vi "Test - Refnum Subtype Enum.vi"() -> ()   [LabVIEW 2020]
uses:
  source/library/oglib_lvdata.lvlib
  source/library/Refnum Subtype Enum.ctl
panel:
  out "30 LabVIEW Class":T1 format="%.0x"
  out "31 Data Value Refnum":T1 format="%.0x"
  out "21 HPT Refnum: Shared Variable Refnum":T1 format="%.0x"
  out "34 TDMS Refnum":T1 format="%.0x"
  out "25 User Event Refnum":T1 format="%.0x"
  out "23 Event Registration Refnum":T1 format="%.0x"
  out "18 Queue Refnum":T1 format="%.0x"
  out "17 Notifier Refnum":T1 format="%.0x"
  out "21 HPT Refnum: DAQmx Global Channel":T1 format="%.0x"
  out "21 HPT Refnum: FieldPoint IO Point":T1 format="%.0x"
  out "14 VISA resource name":T1 format="%.0x"
  out "15 IVI Logical Name":T1 format="%.0x"
  out "21 HPT Refnum: Motion Resource":T1 format="%.0x"
  out "11 IMAQ Session":T1 format="%.0x"
  in  "Motion Resource":refnum<k21>
  in  "FieldPoint IO Point":refnum<k21>
  out "08 VI Server Refnum":T1 format="%.0x"
  out "19 IrDA Refnum":T1 format="%.0x"
  out "31 Bluetooth Refnum":T1 format="%.0x"
  out "24 .NET Refnum":T1 format="%.0x"
  out "27 Event Callback Refnum":T1 format="%.0x"
  out "07 Automation Refnum":T1 format="%.0x"
  out "16 UDP Refnum":T1 format="%.0x"
  out "05 TCP Refnum":T1 format="%.0x"
  out "13 Datasocket Refnum":T1 format="%.0x"
  out "09 Menu Refnum":T1 format="%.0x"
  out "04 Occurence Refnum":T1 format="%.0x"
  out "02 Datalog File Refnum":T1 format="%.0x"
  out "01 Byte Stream File Refnum":T1 format="%.0x"
  out "00 Generic":T1 format="%.0x"
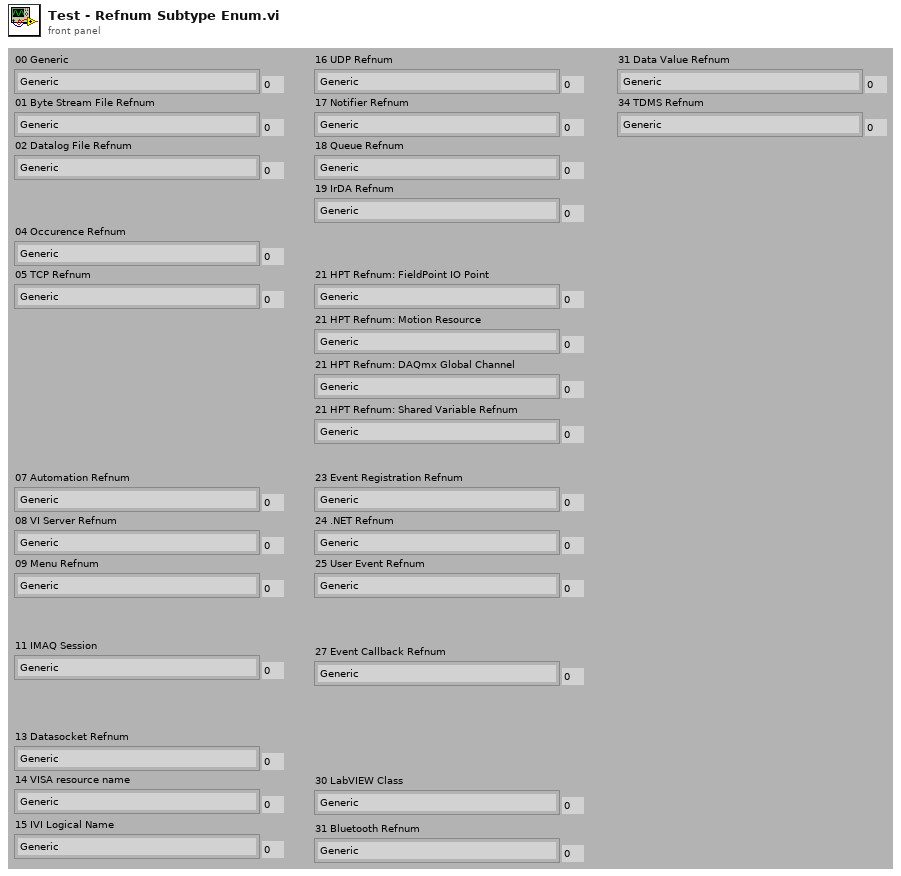
[diagram p1: front panel]
types:
  T1 = typedef "oglib_lvdata.lvlib/Refnum Subtype Enum.ctl" = enum8{"Generic", "Datalog File Refnum", "Byte Stream File Refnum", "Device Refnum", "Occurence Refnum", "TCP Connection Refnum", "VISA Refnum (Obsolete)", "Automation Renum", "VI Server Refnum", "Menu Refnum", "IVI Refnum (Obsolete)", "IMAQ Session", "0x0C", "Datasocket Refnum", "VISA Resource", "IVI Logical Name", "UDP Connection Refnum", "Notifier Refnum", "Queue Refnum", "IrDA Refnum", "Hardware Plugin Refnum", "Hardware Plugin Tag Refnum", "DAQmx Refnum", "Event Registration Refnum", ".NET Refnum", "User Event Refnum", "0x1A", "Event Callback", "0x1C", "0x1D", "LabVIEW Class Instance", "Bluetooth", "Data Value References", "RT FIFO", "TDM Streaming"}
  T2 = typedef "Refnum Subtype Enum.ctl" = enum8{"Generic", "Datalog File Refnum", "Byte Stream File Refnum", "Device Refnum", "Occurence Refnum", "TCP Connection Refnum", "VISA Refnum (Obsolete)", "Automation Renum", "VI Server Refnum", "Menu Refnum", "IVI Refnum (Obsolete)", "IMAQ Session", "0x0C", "Datasocket Refnum", "VISA Resource", "IVI Logical Name", "UDP Connection Refnum", "Notifier Refnum", "Queue Refnum", "IrDA Refnum", "Hardware Plugin Refnum", "Hardware Plugin Tag Refnum", "DAQmx Refnum", "Event Registration Refnum", ".NET Refnum", "User Event Refnum", "0x1A", "Event Callback", "0x1C", "0x1D", "LabVIEW Class Instance", "Bluetooth", "Data Value References", "RT FIFO", "TDM Streaming"}
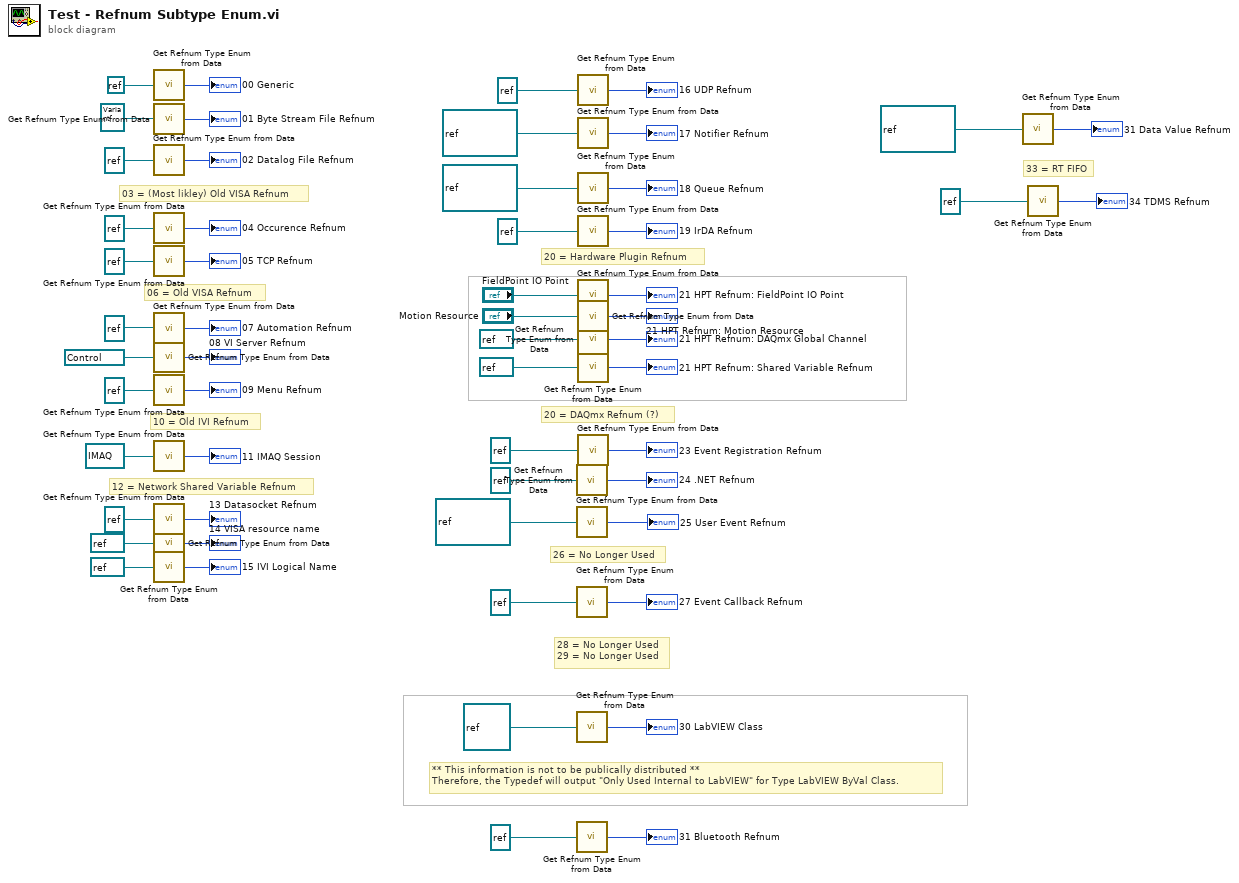
[diagram p0: block diagram]
diagram:
  # "20 = DAQmx Refnum (?)"
  # "20 = Hardware Plugin Refnum"
  # "28 = No Longer Used\n29 = No Longer Used"
  # "26 = No Longer Used"
  # "10 = Old IVI Refnum"
  # "06 = Old VISA Refnum"
  # "03 = (Most likley) Old VISA Refnum"
  # "12 = Network Shared Variable Refnum"
  # "33 = RT FIFO"
  # "** This information is not to be publically distributed **\nTherefore, the Typedef will output \"Only Used Internal to LabVIEW\" for Type LabVIEW ByVal Class."
  n1 = call "Get Refnum Type Enum from Data.vi"("Data"=refnum<k0> refnum) -> ("Refnum Subtype Enum"=→"00 Generic":T2)  [unwired: 4 in]
  n2 = call "Get Refnum Type Enum from Data.vi"("Data"=refnum<k1> refnum ("refnum out")) -> ("Refnum Subtype Enum"=→"01 Byte Stream File Refnum":T2)  [unwired: 4 in]
  n3 = call "Get Refnum Type Enum from Data.vi"("Data"=refnum<file> refnum ("refnum")) -> ("Refnum Subtype Enum"=→"02 Datalog File Refnum":T2)  [unwired: 4 in]
  n4 = call "Get Refnum Type Enum from Data.vi"("Data"=refnum<k4> refnum ("occurrence")) -> ("Refnum Subtype Enum"=→"04 Occurence Refnum":T2)  [unwired: 4 in]
  n5 = call "Get Refnum Type Enum from Data.vi"("Data"=refnum<k5> refnum ("TCP Network Connection Refnum")) -> ("Refnum Subtype Enum"=→"05 TCP Refnum":T2)  [unwired: 4 in]
  n6 = call "Get Refnum Type Enum from Data.vi"("Data"=refnum<k7> refnum ("Automation Refnum")) -> ("Refnum Subtype Enum"=→"07 Automation Refnum":T2)  [unwired: 4 in]
  n7 = call "Get Refnum Type Enum from Data.vi"("Data"=refnum<vi> refnum ("Ctl Refnum")) -> ("Refnum Subtype Enum"=→"08 VI Server Refnum":T2)  [unwired: 4 in]
  n8 = call "Get Refnum Type Enum from Data.vi"("Data"=refnum<k9> refnum ("Menu Refnum")) -> ("Refnum Subtype Enum"=→"09 Menu Refnum":T2)  [unwired: 4 in]
  n9 = call "Get Refnum Type Enum from Data.vi"("Data"=refnum<k11> refnum ("IMAQ Session")) -> ("Refnum Subtype Enum"=→"11 IMAQ Session":T2)  [unwired: 4 in]
  n10 = call "Get Refnum Type Enum from Data.vi"("Data"=refnum<k13> refnum ("DataSocket Refnum")) -> ("Refnum Subtype Enum"=→"13 Datasocket Refnum":T2)  [unwired: 4 in]
  n11 = call "Get Refnum Type Enum from Data.vi"("Data"=refnum<visa-resource-name> refnum ("VISA resource name")) -> ("Refnum Subtype Enum"=→"14 VISA resource name":T2)  [unwired: 4 in]
  n12 = call "Get Refnum Type Enum from Data.vi"("Data"=refnum<k15> refnum ("IVI Logical Name")) -> ("Refnum Subtype Enum"=→"15 IVI Logical Name":T2)  [unwired: 4 in]
  n13 = call "Get Refnum Type Enum from Data.vi"("Data"=refnum<k24> refnum (".NET Refnum")) -> ("Refnum Subtype Enum"=→"24 .NET Refnum":T2)  [unwired: 4 in]
  n14 = call "Get Refnum Type Enum from Data.vi"("Data"=refnum<user-event> refnum ("user event out")) -> ("Refnum Subtype Enum"=→"25 User Event Refnum":T2)  [unwired: 4 in]
  n15 = call "Get Refnum Type Enum from Data.vi"("Data"=refnum<k27> refnum ("Event Callback")) -> ("Refnum Subtype Enum"=→"27 Event Callback Refnum":T2)  [unwired: 4 in]
  n16 = call "Get Refnum Type Enum from Data.vi"("Data"=refnum<class> refnum ("LabVIEW Object")) -> ("Refnum Subtype Enum"=→"30 LabVIEW Class":T2)  [unwired: 4 in]
  n17 = call "Get Refnum Type Enum from Data.vi"("Data"=refnum<k31> refnum ("Bluetooth Refnum")) -> ("Refnum Subtype Enum"=→"31 Bluetooth Refnum":T2)  [unwired: 4 in]
  n18 = call "Get Refnum Type Enum from Data.vi"("Data"=refnum<k16> refnum ("UDP Network Connection Refnum")) -> ("Refnum Subtype Enum"=→"16 UDP Refnum":T2)  [unwired: 4 in]
  n19 = call "Get Refnum Type Enum from Data.vi"("Data"=refnum<notifier> refnum ("notifier out")) -> ("Refnum Subtype Enum"=→"17 Notifier Refnum":T2)  [unwired: 4 in]
  n20 = call "Get Refnum Type Enum from Data.vi"("Data"=refnum<queue> refnum ("queue out")) -> ("Refnum Subtype Enum"=→"18 Queue Refnum":T2)  [unwired: 4 in]
  n21 = call "Get Refnum Type Enum from Data.vi"("Data"=refnum<k19> refnum ("IrDA Refnum")) -> ("Refnum Subtype Enum"=→"19 IrDA Refnum":T2)  [unwired: 4 in]
  n22 = call "Get Refnum Type Enum from Data.vi"("Data"="FieldPoint IO Point") -> ("Refnum Subtype Enum"=→"21 HPT Refnum: FieldPoint IO Point":T2)  [unwired: 4 in]
  n23 = call "Get Refnum Type Enum from Data.vi"("Data"="Motion Resource") -> ("Refnum Subtype Enum"=→"21 HPT Refnum: Motion Resource":T2)  [unwired: 4 in]
  n24 = call "Get Refnum Type Enum from Data.vi"("Data"=refnum<k21> refnum ("DAQmx Global Channel")) -> ("Refnum Subtype Enum"=→"21 HPT Refnum: DAQmx Global Channel":T2)  [unwired: 4 in]
  n25 = call "Get Refnum Type Enum from Data.vi"("Data"=refnum<k21> refnum ("shared variable refnum out")) -> ("Refnum Subtype Enum"=→"21 HPT Refnum: Shared Variable Refnum":T2)  [unwired: 4 in]
  n26 = call "Get Refnum Type Enum from Data.vi"("Data"=refnum<event-registration> refnum ("event registration refnum")) -> ("Refnum Subtype Enum"=→"23 Event Registration Refnum":T2)  [unwired: 4 in]
  n27 = call "Get Refnum Type Enum from Data.vi"("Data"=refnum<data-value> refnum ("data value reference")) -> ("Refnum Subtype Enum"=→"31 Data Value Refnum":T2)  [unwired: 4 in]
  n28 = call "Get Refnum Type Enum from Data.vi"("Data"=refnum<k34> refnum ("tdms file out")) -> ("Refnum Subtype Enum"=→"34 TDMS Refnum":T2)  [unwired: 4 in]
